vi "remote.Property Node Read Core.vi"(8 "error in (no error)":errorcluster, 10 "property":string, 11 "SLSC Remote in":refnum<class "SLSC Interface.lvclass">) -> (0 "error out":errorcluster, 2 "value":refnum<class "JSON Null.lvclass">, 3 "SLSC Remote out":refnum<class "SLSC Interface.lvclass">)   [LabVIEW 2016, in "SLSC Interface.lvclass"]
uses:
  SLSC Interface Class/SLSC Interface.lvclass
  <vilib>/NI/JSON Support for LabVIEW/JSON Data Classes/JSON Datatype/JSON Null.lvclass
  SLSC Interface Class/SLSC Interface.lvclass/SLSC Interface.ctl
  SLSC Interface Class/Read client handle.vi
  SLSC Interface Class/Read URL.vi
  <vilib>/NI/JSON Support for LabVIEW/JSON Data Classes/JSON Object/JSON Object.lvclass
  C:/Program Files (x86)/National Instruments/LabVIEW 2016/vi.lib/NI/JSON Support for LabVIEW/JSON Data Classes/JSON Datatype/JSON Null.lvclass
  SLSC Interface Class/Read session.vi
  <vilib>/NI/JSON Support for LabVIEW/JSON Data Classes/JSON Object/New JSON Object (Empty).vi
  <vilib>/NI/JSON Support for LabVIEW/JSON Data Classes/JSON Object/Insert Key Value Pair (Single String).vi
  <vilib>/NI/NI JSONRPC Server Framework/Classes/Server/Format Client Request (Auto-Increment).vi
  <vilib>/httpClient/POSTBuffer.vi
  <vilib>/NI/NI JSONRPC Server Framework/Classes/Server/Parse Response (Object).vi
  <vilib>/NI/JSON Support for LabVIEW/JSON Data Classes/JSON Object/Get Value (JSON).vi
  <vilib>/NI/NI JSONRPC Server Framework/Classes/Server/JSONRPC Server.lvclass
  <vilib>/httpClient/LabVIEWHTTPClient.lvlib
  <vilib>/NI/JSON Support for LabVIEW/JSON Data Classes/JSON Helper/JSON Helper.lvclass
  C:/Program Files (x86)/National Instruments/LabVIEW 2016/vi.lib/NI/JSON Support for LabVIEW/JSON Data Classes/JSON Structured Type/JSON Structure.lvclass
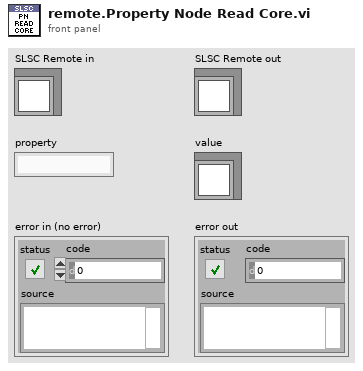
[diagram p1: front panel]
types:
  T1 = typedef "LabVIEWHTTPClient.lvlib/ClientHandle.ctl" = refnum<k1>
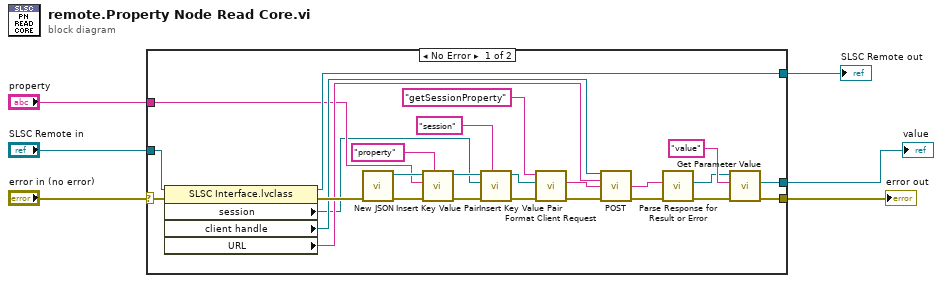
[diagram p0: block diagram]
diagram:
  n1 = case shown="No Error" "error in (no error)" {
    selector: "error in (no error)" -> [w30 w33]
    tunnel: "SLSC Remote in" -> [w32 w34]
    tunnel: [w31 w34] -> w3
    tunnel: [w15 w33] -> w4
    tunnel: [w16 _] -> w1
    tunnel: "property" -> [w9 _]
    frame No Error {
      n2 = property class="SLSC Interface.lvclass"(reference=w32, error in=w30) -> (reference out=w31:refnum<class "SLSC Interface.lvclass">, error out=w29:errorcluster, "session"=w8:refnum<k21>, "client handle"=w22:T1, "URL"=w21:string)
      n3 = call-poly <vilib>:"New JSON.vi"("error in (no error)"=w29) -> ("error out"=w28:errorcluster, "JSON Object out"=w12:refnum<class "JSON Object.lvclass">)  [unwired: 9 in]
      n4 = call-poly <vilib>:"Insert Key Value Pair.vi"("key"="property" ("Name"), "error in (no error)"=w28, "value"=w9, "JSON Object in"=w12) -> ("error out"=w25:errorcluster, "JSON Object out"=w11:refnum<class "JSON Object.lvclass">)  [unwired: 5 in, 1 out]
      n5 = call-poly <vilib>:"Insert Key Value Pair.vi"("key"="session" ("Name"), "error in (no error)"=w25, "value"=w8, "JSON Object in"=w11) -> ("error out"=w23:errorcluster, "JSON Object out"=w24:refnum<class "JSON Object.lvclass">)  [unwired: 5 in, 1 out]
      n6 = call-poly <vilib>:"Format Client Request.vi"("error in (no error)"=w23, "JSON in"=w24, "method"="getSessionProperty") -> ("error out"=w20:errorcluster, "Request String"=w26:string)  [unwired: 7 in]
      n7 = call-poly <vilib>:"POST.vi"("client handle"=w22, "url"=w21, "buffer"=w26, "error in (no error)"=w20) -> ("body"=w19:string, "error out"=w18:errorcluster)  [unwired: 8 in, 2 out]
      n8 = call-poly <vilib>:"Parse Response for Result or Error.vi"("error in"=w18, "Response String In"=w19) -> ("error out"=w10:errorcluster, "JSON Array"=w7:refnum<class "JSON Object.lvclass">)  [unwired: 7 in, 1 out]
      n9 = call-poly <vilib>:"Get Parameter Value.vi"("error in (no error)"=w10, "key"="value" ("Parameter Name"), "JSON Object in"=w7) -> ("error out"=w15:errorcluster, "value"=w16:refnum<class "JSON Null.lvclass">)  [unwired: 7 in]
    }
    frame Error {
    }
  }
  "error out" <- w4
  "SLSC Remote out" <- w3
  "value" <- w1
